vi "Stepping X.vi"(7 "Microstep size":T1(ring), 8 "error in (no error)":errorcluster, 9 "Speed":u32=5, 10 "Direction":bool, 11 "Enable":bool) -> (0 "error out":errorcluster)   [LabVIEW 2017]
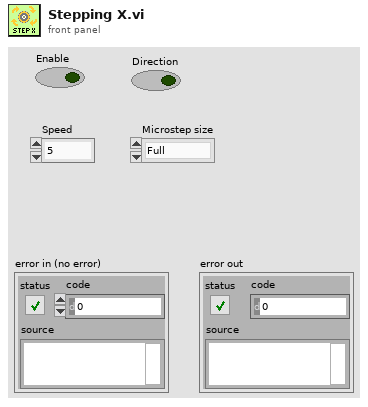
[diagram p1: front panel]
types:
  T1 = enum16{"Full", "Half", "Quarter", "Eighth", "Sixteenth"}
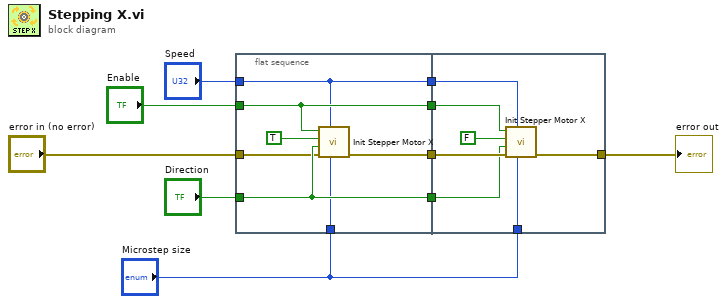
[diagram p0: block diagram]
diagram:
  n1 = flat-sequence {
    tunnel: [w17] -> w10
    tunnel: [w16] -> w9
    tunnel: "Enable" -> [w16]
    tunnel: "Speed" -> [w15]
    tunnel: [w15] -> w8
    tunnel: "Direction" -> [w13]
    tunnel: [w13] -> w7
    tunnel: "error in (no error)" -> [w12]
    tunnel: "Microstep size" -> [w11]
    tunnel: w10 -> [w24]
    tunnel: w9 -> [w23]
    tunnel: w8 -> [w22]
    tunnel: w7 -> [w20]
    tunnel: [w19] -> w5
    tunnel: "Microstep size" -> [w18]
    frame #0 {
      n2 = call "Init Stepper Motor X.vi"("Microstep size"=w11, "Speed"=w15, "error in (no error)"=w12, "Direction (C/DIO4 (DIO4))"=w13, "Step (C/DIO3 (DIO3))"=TRUE, "Enable (C/DIO2 (DIO2))"=w16) -> ("error out"=w17:errorcluster)  [unwired: 5 in]
    }
    frame #1 {
      n3 = call "Init Stepper Motor X.vi"("Microstep size"=w18, "Speed"=w22, "error in (no error)"=w24, "Direction (C/DIO4 (DIO4))"=w20, "Step (C/DIO3 (DIO3))"=FALSE, "Enable (C/DIO2 (DIO2))"=w23) -> ("error out"=w19:errorcluster)  [unwired: 5 in]
    }
  }
  "error out" <- w5
